vi "模块配置读取.vi"(8 "error in (no error)":errorcluster caption="错误输入（无错误）") -> (0 "error out":errorcluster caption="错误输出")   [LabVIEW 2016, in "斯坦道总磷.lvlib"]
uses:
  <vilib>/Utility/config.llb/NI_LVConfig.lvlib
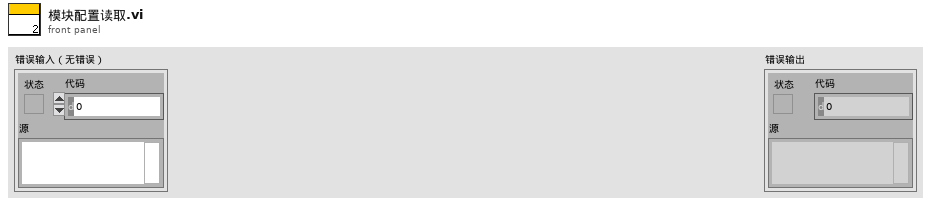
[diagram p1: front panel]
types:
  T1 = typedef "NI_LVConfig.lvlib/Config Data RefNum.ctl" = refnum<k1>
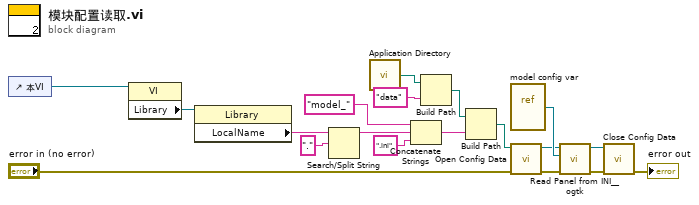
[diagram p0: block diagram]
diagram:
  n1 = control-ref of="本VI"() -> (w8:refnum<vi>)
  n2 = property class="VI"(reference=w8) -> ("Library"=w9:refnum<vi>)  [unwired: 1 in, 2 out]
  n3 = property class="Library"(reference=w9) -> ("LocalName"=w7:string)  [unwired: 1 in, 2 out]
  n4 = Search/Split String(string=w7, search string/char (-)="." ("搜索字符串/字符(-)")) -> (substring before match=w5:string)  [unwired: 1 in, 2 out]
  n5 = call <vilib>:"Application Directory.vi"() -> ("Application Directory"=w11:path)
  n6 = Concatenate Strings("model_" ("字符串"), w5, ".ini" ("字符串")) -> (w4:string)
  n7 = Build Path(base path=w11, name or relative path="data" ("名称或相对路径")) -> (appended path=w10:path)
  n8 = Build Path(base path=w10, name or relative path=w4) -> (appended path=w1:path)
  n9 = vi-ref "model config var.vi"() -> (w16:refnum<vi>)
  n10 = call <vilib>:"Open Config Data.vi"("error in (no error)"="error in (no error)", "configuration file path"=w1) -> ("error out"=w18:errorcluster, "refnum"=w15:T1)  [unwired: 7 in, 1 out]
  n11 = call <userlib>:"Read Panel from INI__ogtk.vi"("error in (no error)"=w18, "VI ref"=w16, "refnum"=w15) -> ("error out"=w19:errorcluster, "refnum out"=w17:T1)  [unwired: 7 in]
  n12 = call <vilib>:"Close Config Data.vi"("error in (no error)"=w19, "refnum"=w17) -> ("error out"=→"error out":errorcluster)  [unwired: 8 in, 1 out]
